vi "Configure Jitter Free Trigger.vi"(8 "error in (no error)":errorcluster, 10 "Enable Jitter Free Trigger (T: Enable)":bool=TRUE, 11 "VISA resource name":refnum<visa-resource-name>) -> (0 "error out":errorcluster, 3 "VISA resource name out":refnum<visa-resource-name>)   [LabVIEW 2017, in "Agilent 2000 3000 X-Series.lvlib"]
doc: "Disables or enables the Jitter-Free Trigger option\n\n<b>Note:</b>\nThis VI is specific to the 6000-X Series oscilloscopes. These features are not available on other models. If the instrument is not configured correctly prior to running this VI a -221, \"Settings conflict\" error will be produced. This feature is only available in certain modes."
uses:
  Agilent 2000 3000 X-Series.lvlib
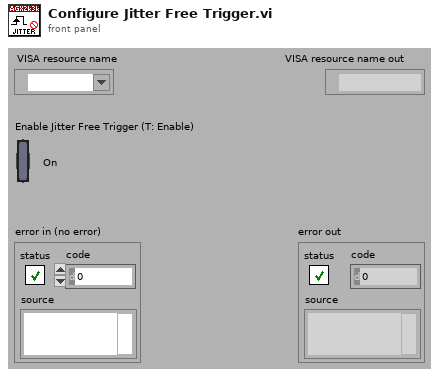
[diagram p1: front panel]
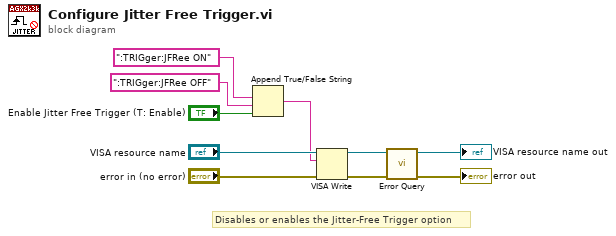
[diagram p0: block diagram]
diagram:
  # "Disables or enables the Jitter-Free Trigger option"
  n1 = Append True/False String(1:"Enable Jitter Free Trigger (T: Enable)", 2:":TRIGger:JFRee OFF", 3:":TRIGger:JFRee ON") -> (0:w1:string)  [unwired: 1 in]
  n2 = VISA Write(VISA resource name="VISA resource name", write buffer=w1, error in (no error)="error in (no error)") -> (VISA resource name out=w6:refnum<visa-resource-name>, error out=w5:errorcluster)  [unwired: 1 out]
  n3 = call "Error Query.vi"("error in (no error)"=w5, "VISA resource name"=w6) -> ("error out"=→"error out":errorcluster, "VISA resource name out"=→"VISA resource name out":refnum<visa-resource-name>)  [unwired: 8 out]
